vi "StrListDetailHandle.vi"(4 "Text":string, 5 "ErrorIn":errorcluster, 6 "StrIndex":i32, 7 "MethodChoose":i32) -> (1 "ErrorOut":errorcluster, 2 "ItemNames":string[](array[string]), 3 "ItemSymbols":i32[](array[numeric]))   [LabVIEW 2023]
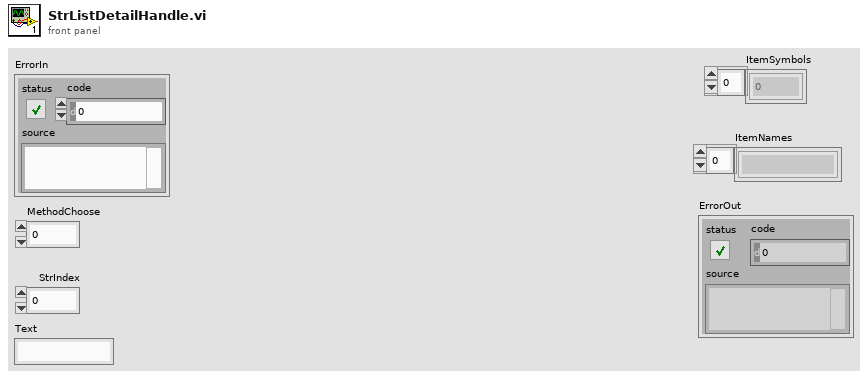
[diagram p1: front panel]
types:
  T1 = enum16{"open", "replace", "create", "open or create", "replace or create", "replace or create with confirmation"}
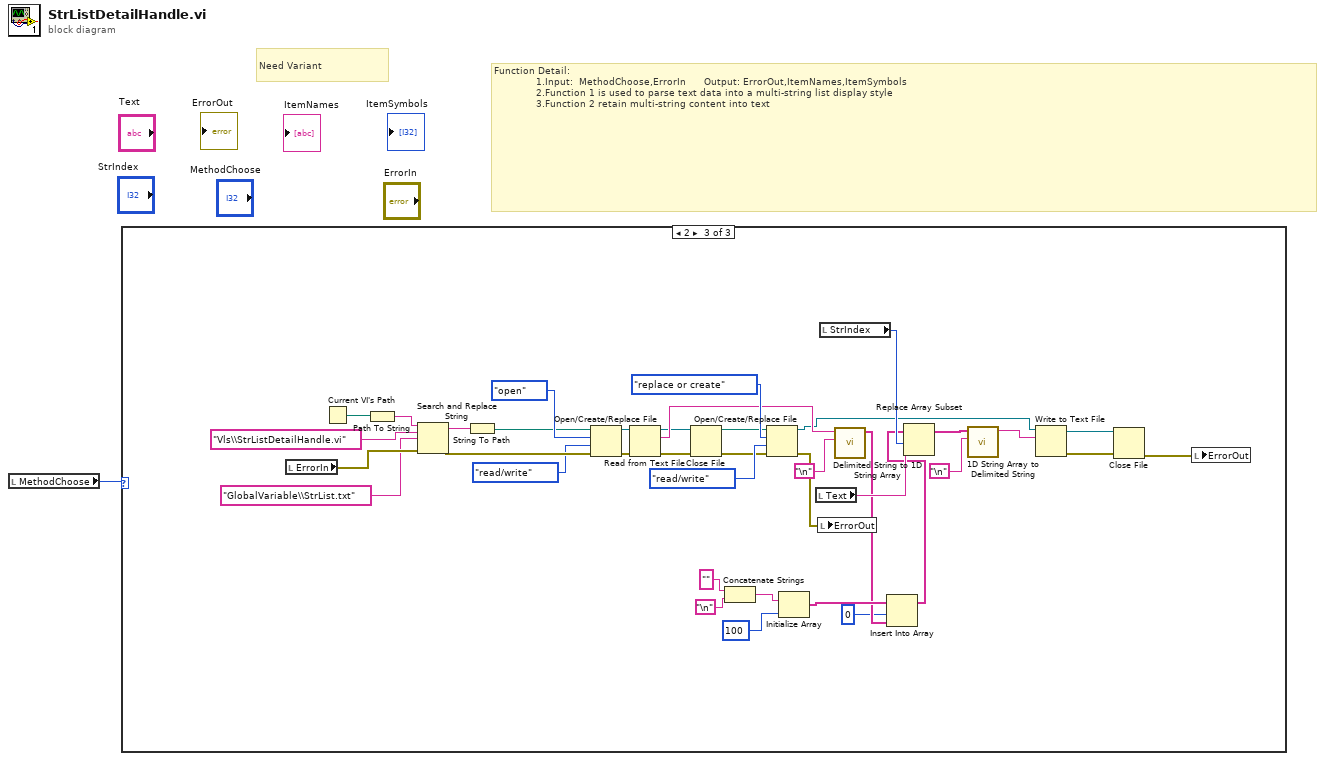
[diagram p0: block diagram]
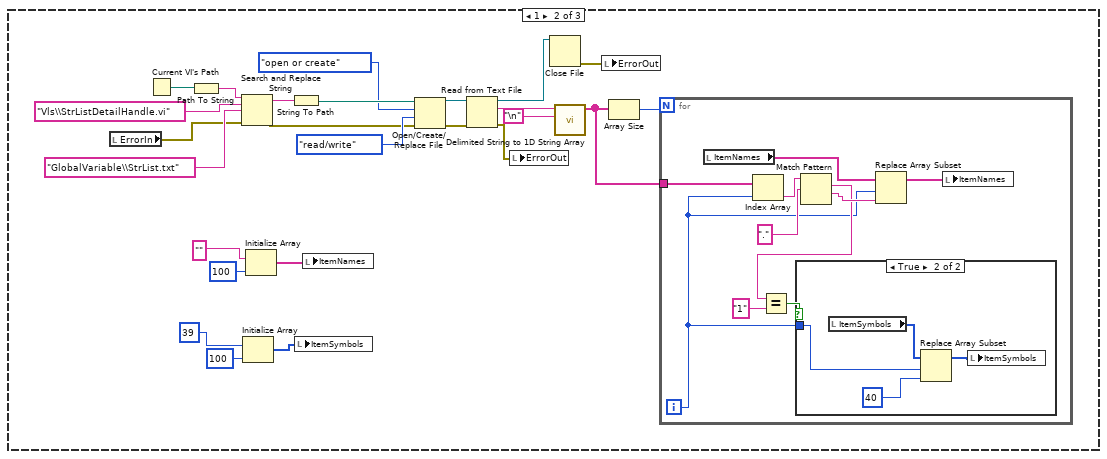
[diagram p3: hidden frame]
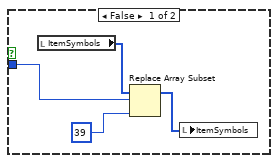
[diagram p4: hidden frame]
diagram:
  # "Function Detail:\n              1.Input:  MethodChoose,ErrorIn      Output: ErrorOut,ItemNames,ItemSymbols\n              2.Function 1 is used to parse text data into a multi-string list display style\n              3.Function 2 retain multi-string content into text"
  # "Need Variant"
  n1 = local read "MethodChoose"() -> (w1:i32)
  n2 = case shown="2" w1 {
    frame 0, Default {
    }
    frame 1 {
      n3 = local read "ErrorIn"() -> (w13:errorcluster)
      n4 = Current VI's Path() -> (path=w21:path)
      n5 = Path To String(path=w21) -> (string=w22:string)
      n6 = Search and Replace String(input string=w22, search string="Vls\\StrListDetailHandle.vi", replace string="GlobalVariable\\StrList.txt" ("replace string (\"\")"), error in=w13) -> (result string=w23:string, error out=w12:errorcluster)  [unwired: 4 in, 2 out]
      n7 = Initialize Array(39, 100 ("dimension size")) -> (w2:i32[])
      n8 = Initialize Array("", 100 ("dimension size")) -> (w6:string[])
      n9 = String To Path(string=w23) -> (path=w24:path)
      n10 = local write "ItemSymbols"(w2) -> ()
      n11 = local write "ItemNames"(w6) -> ()
      n12 = Open/Create/Replace File(file path (use dialog)=w24, error in=w12, operation (0:open)=T1."open or create", access (0:read/write)=enum16{"read/write", "read-only", "write-only"}."read/write") -> (refnum out=w25:refnum<file>, error out=w11:errorcluster)  [unwired: 2 in, 1 out]
      n13 = Read from Text File(file (use dialog)=w25, error in=w11) -> (refnum out=w9:refnum<file>, text=w26:string, error out=w10:errorcluster)  [unwired: 2 in, 1 out]
      n14 = local write "ErrorOut"(w10) -> ()
      n15 = Close File(refnum=w9) -> (error out=w8:errorcluster)  [unwired: 1 in, 1 out]
      n16 = call <vilib>:"Delimited String to 1D String Array.vi"("delimiter"="\n", "delimited string"=w26) -> ("string array"=w14:string[])  [unwired: 9 in]
      n17 = local write "ErrorOut"(w8) -> ()
      n18 = Array Size(array=w14) -> (size(s)=w15:i32)
      n19 = for {
        N: w15 -> [_]
        tunnel: w14 -> [w36]
        i -> [w29]
        n20 = local read "ItemNames"() -> (w27:string[])
        n21 = Index Array(array=w36, index=w29) -> (element=w35:string)
        n22 = Match Pattern(string=w35, regular expression=".") -> (match substring=w31:string, after substring=w33:string)  [unwired: 1 in, 2 out]
        n23 = Equal?(x=w31, y="1") -> (x = y?=w32:bool)
        n24 = case shown="True" w32 {
          tunnel: w29 -> [w39 w44]
          frame False {
            n25 = local read "ItemSymbols"() -> (w37:i32[])
            n26 = Replace Array Subset(array=w37, new element=39 ("new element/subarray"), index=w39) -> (w38:i32[])
            n27 = local write "ItemSymbols"(w38) -> ()
          }
          frame True {
            n28 = local read "ItemSymbols"() -> (w41:i32[])
            n29 = Replace Array Subset(array=w41, new element=40 ("new element/subarray"), index=w44) -> (w42:i32[])
            n30 = local write "ItemSymbols"(w42) -> ()
          }
        }
        n31 = Replace Array Subset(array=w27, new element=w33, index=w29) -> (w28:string[])
        n32 = local write "ItemNames"(w28) -> ()
      }
    }
    frame 2 {
      n33 = local read "ErrorIn"() -> (w79:errorcluster)
      n34 = Current VI's Path() -> (path=w80:path)
      n35 = Path To String(path=w80) -> (string=w81:string)
      n36 = Search and Replace String(input string=w81, search string="Vls\\StrListDetailHandle.vi", replace string="GlobalVariable\\StrList.txt" ("replace string (\"\")"), error in=w79) -> (result string=w82:string, error out=w78:errorcluster)  [unwired: 4 in, 2 out]
      n37 = String To Path(string=w82) -> (path=w62:path)
      n38 = Open/Create/Replace File(file path (use dialog)=w62, error in=w78, operation (0:open)=T1."open", access (0:read/write)=enum16{"read/write", "read-only", "write-only"}."read/write") -> (refnum out=w73:refnum<file>, error out=w72:errorcluster)  [unwired: 2 in, 1 out]
      n39 = Read from Text File(file (use dialog)=w73, error in=w72) -> (refnum out=w56:refnum<file>, text=w59:string, error out=w57:errorcluster)  [unwired: 2 in, 1 out]
      n40 = Close File(refnum=w56, error in=w57) -> (path=w55:path, error out=w54:errorcluster)
      n41 = Concatenate Strings("" ("Text"), "\n") -> (w50:string)
      n42 = Open/Create/Replace File(file path (use dialog)=w55, error in=w54, operation (0:open)=T1."replace or create", access (0:read/write)=enum16{"read/write", "read-only", "write-only"}."read/write") -> (refnum out=w53:refnum<file>, error out=w58:errorcluster)  [unwired: 2 in, 1 out]
      n43 = Initialize Array(w50, 100 ("dimension size")) -> (w48:string[])
      n44 = local read "Text"() -> (w69:string)
      n45 = local write "ErrorOut"(w58) -> ()
      n46 = local read "StrIndex"() -> (w70:i32)
      n47 = call <vilib>:"Delimited String to 1D String Array.vi"("delimiter"="\n", "delimited string"=w59) -> ("string array"=w47:string[])  [unwired: 9 in]
      n48 = Insert Into Array(array=w48, index=0, new element=w47) -> (w45:string[])
      n49 = Replace Array Subset(array=w45, new element=w69, index=w70) -> (w68:string[])
      n50 = call <vilib>:"1D String Array to Delimited String.vi"("delimiter"="\n", "string array"=w68) -> ("delimited string"=w66:string)  [unwired: 9 in]
      n51 = Write to Text File(file (use dialog)=w53, text=w66) -> (refnum out=w64:refnum<file>, error out=w65:errorcluster)  [unwired: 2 in, 1 out]
      n52 = Close File(refnum=w64, error in=w65) -> (error out=w63:errorcluster)  [unwired: 1 out]
      n53 = local write "ErrorOut"(w63) -> ()
    }
  }
